vi "Train assignment.vi"() -> ()   [LabVIEW 2018]
panel:
  out "Berth Allocated":string
  in  "Berth Number    Number":dbl
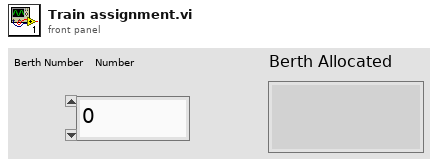
[diagram p1: front panel]
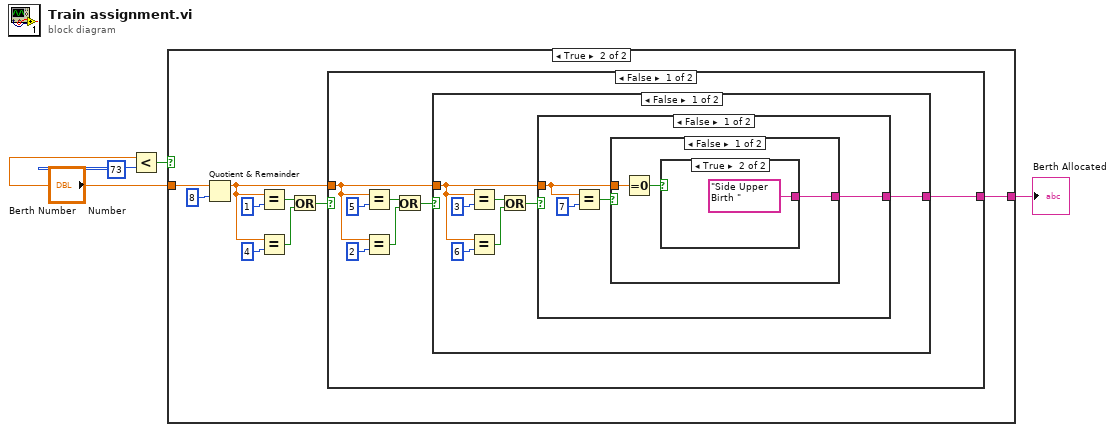
[diagram p0: block diagram]
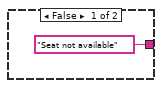
[diagram p2: hidden frame]
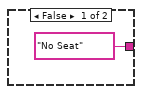
[diagram p3: hidden frame]
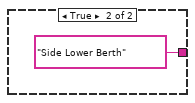
[diagram p4: hidden frame]
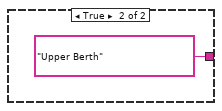
[diagram p5: hidden frame]
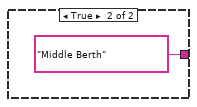
[diagram p6: hidden frame]
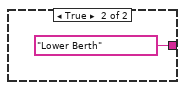
[diagram p7: hidden frame]
diagram:
  n1 = Less?(x="Berth Number    Number", y=73) -> (x < y?=w3:bool)
  n2 = case shown="True" w3 {
    tunnel: "Berth Number    Number" -> [_ w14]
    tunnel: ["Seat not available" w6] -> w1
    frame False {
    }
    frame True {
      n3 = Quotient & Remainder(x=w14, y=8) -> (x-y*floor(x/y)=w7:dbl)  [unwired: 1 out]
      n4 = Equal?(x=w7, y=1) -> (x = y?=w10:bool)
      n5 = Equal?(x=w7, y=4) -> (x = y?=w9:bool)
      n6 = Or(x=w10, y=w9) -> (x .or. y?=w8:bool)
      n7 = case shown="False" w8 {
        tunnel: w7 -> [w16 _]
        tunnel: [w15 "Lower Berth"] -> w6
        frame False {
          n8 = Equal?(x=w16, y=5) -> (x = y?=w19:bool)
          n9 = Equal?(x=w16, y=2) -> (x = y?=w18:bool)
          n10 = Or(x=w19, y=w18) -> (x .or. y?=w17:bool)
          n11 = case shown="False" w17 {
            tunnel: w16 -> [w23 _]
            tunnel: [w22 "Middle Berth"] -> w15
            frame False {
              n12 = Equal?(x=w23, y=3) -> (x = y?=w26:bool)
              n13 = Equal?(x=w23, y=6) -> (x = y?=w25:bool)
              n14 = Or(x=w26, y=w25) -> (x .or. y?=w24:bool)
              n15 = case shown="False" w24 {
                tunnel: w23 -> [w31 _]
                tunnel: [w29 "Upper Berth"] -> w22
                frame False {
                  n16 = Equal?(x=w31, y=7) -> (x = y?=w30:bool)
                  n17 = case shown="False" w30 {
                    tunnel: w31 -> [w35 _]
                    tunnel: [w33 "Side Lower Berth"] -> w29
                    frame False {
                      n18 = Equal To 0?(x=w35) -> (x = 0?=w34:bool)
                      n19 = case shown="True" w34 {
                        tunnel: ["No Seat" "Side Upper Birth "] -> w33
                        frame False {
                        }
                        frame True {
                        }
                      }
                    }
                    frame True {
                    }
                  }
                }
                frame True {
                }
              }
            }
            frame True {
            }
          }
        }
        frame True {
        }
      }
    }
  }
  "Berth Allocated" <- w1
